vi "Translation_Times.vi"(9 "Scalar":dbl, 11 "In Translation":T1) -> (3 "Out Translation":T1)   [LabVIEW 2019, in "Trajectory_Library.lvlib"]
doc: "Multiplies the translation by a scalar and returns the new translation.\n\nFor example, Translation2d{2.0, 2.5} * 2 = Translation2d{4.0, 5.0}\n\nParameters:\n - In Translation - This translation data structure\n - scalar - The value to multiply the translation by\n\nResult:\n - Out Translation - The resulting translation"
uses:
  Trajectory_Library.lvlib
  TRANSLATION2D.ctl
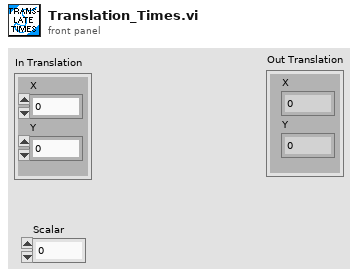
[diagram p1: front panel]
types:
  T1 = typedef "Trajectory_Library.lvlib/TRANSLATION2D.ctl" = cluster{"X":dbl, "Y":dbl}
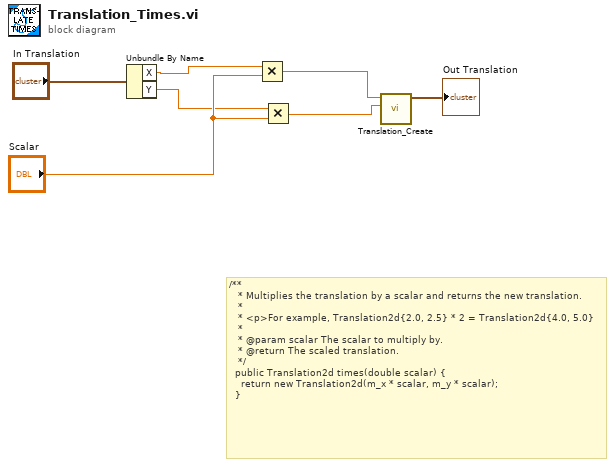
[diagram p0: block diagram]
diagram:
  # "/**\n   * Multiplies the translation by a scalar and returns the new translation.\n   *\n   * <p>For example, Translation2d{2.0, 2.5} * 2 = Translation2d{4.0, 5.0}\n   *\n   * @param scalar The scalar to multiply by.\n   * @return The scaled translation.\n   */\n  public Translation2d times(double scalar) {\n    return new Translation2d(m_x * scalar, m_y * scalar);\n  }"
  n1 = Unbundle By Name("In Translation") -> ("X"=w4:dbl, "Y"=w3:dbl)
  n2 = Multiply(x=w4, y="Scalar") -> (x*y=w2:dbl)
  n3 = Multiply(x=w3, y="Scalar") -> (x*y=w1:dbl)
  n4 = call "Translation_Create.vi"("Y"=w1, "X"=w2) -> ("TRANSLATION"=→"Out Translation":T1)  [unwired: 9 in]
